vi "Remove NaN-containing Pairs.vi"(8 "Error In":errorcluster, 9 "Y Array in":dbl[](array[numeric]), 10 "Elements to remove (NaN)":dbl[](array[numeric])=[nan], 11 "X Array in":dbl[](array[numeric])) -> (0 "Error Out":errorcluster, 1 "Y Array out":dbl[](array[numeric]), 2 "# X elts deleted":i32, 3 "X Array out":dbl[](array[numeric]), 4 "Deleted Elts Indices":i32[](array[numeric]))   [LabVIEW 2021, in "Arrays.lvlib"]
uses:
  Arrays.lvlib
  <userlib>/_OpenG.lib/array/array.llb/Search 1D Array (DBL)__ogtk.vi
  <userlib>/_OpenG.lib/array/array.llb/Sort 1D Array (I32)__ogtk.vi
  <userlib>/_OpenG.lib/array/array.llb/Remove Duplicates from 1D Array (I32)__ogtk.vi
  <userlib>/_OpenG.lib/array/array.llb/Delete Elements from 1D Array (DBL)__ogtk.vi
  <userlib>/_OpenG.lib/array/array.llb/openg_array.lvlib
panel:
  out "# Y elts deleted":i32
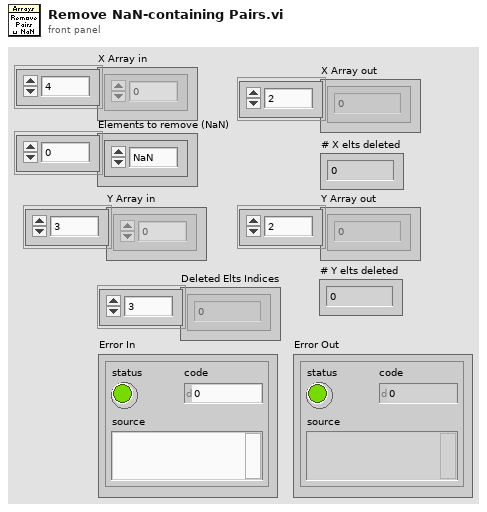
[diagram p1: front panel]
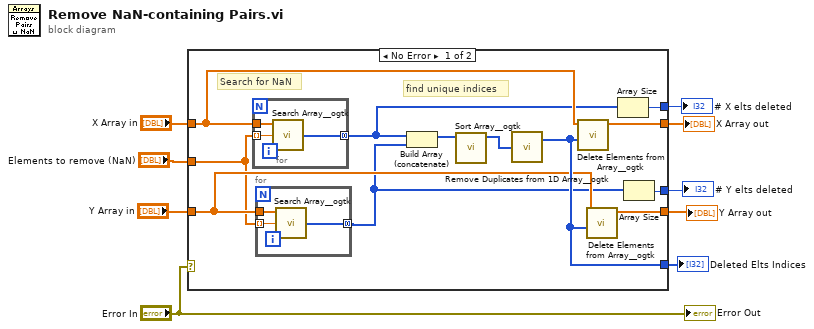
[diagram p0: block diagram]
diagram:
  n1 = case shown="No Error" "Error In" {
    tunnel: "X Array in" -> [w15 w29]
    tunnel: [w20 w29] -> w8
    tunnel: "Y Array in" -> [w13 w28]
    tunnel: [w19 w28] -> w6
    tunnel: [w18 _] -> w5
    tunnel: [w17 _] -> w4
    tunnel: [w16 _] -> w2
    tunnel: "Elements to remove (NaN)" -> [w12 _]
    frame No Error {
      # "find unique indices"
      # "Search for NaN"
      n2 = for {
        tunnel: w15 -> [w27]
        tunnel: [w25] -> w11 mode=concatenating
        tunnel: w12 -> [w26] mode=indexing
        n3 = call-poly <userlib>:"Search Array__ogtk.vi"("Array"=w27, "Element Data"=w26) -> ("Indices of Elements"=w25:i32[])  [unwired: 7 in]
      }
      n4 = for {
        tunnel: w13 -> [w24]
        tunnel: [w22] -> w10 mode=concatenating
        tunnel: w12 -> [w23] mode=indexing
        n5 = call-poly <userlib>:"Search Array__ogtk.vi"("Array"=w24, "Element Data"=w23) -> ("Indices of Elements"=w22:i32[])  [unwired: 7 in]
      }
      n6 = Build Array (concatenate)(w11, w10) -> (w14:i32[])
      n7 = call-poly <userlib>:"Sort Array__ogtk.vi"("Array in"=w14) -> ("Sorted Array out"=w21:i32[])  [unwired: 9 in, 1 out]
      n8 = call-poly <userlib>:"Remove Duplicates from 1D Array__ogtk.vi"("Input Array"=w21) -> ("Output Array"=w16:i32[])  [unwired: 1 out]
      n9 = call-poly <userlib>:"Delete Elements from Array__ogtk.vi"("indices"=w16, "array"=w15) -> ("array w/ subset deleted"=w20:dbl[])  [unwired: 8 in, 1 out]
      n10 = call-poly <userlib>:"Delete Elements from Array__ogtk.vi"("indices"=w16, "array"=w13) -> ("array w/ subset deleted"=w19:dbl[])  [unwired: 8 in, 1 out]
      n11 = Array Size(array=w11) -> (size(s)=w18:i32)
      n12 = Array Size(array=w10) -> (size(s)=w17:i32)
    }
    frame Error {
    }
  }
  "Y Array out" <- w6
  "X Array out" <- w8
  "# X elts deleted" <- w5
  "# Y elts deleted" <- w4
  "Deleted Elts Indices" <- w2
  "Error Out" <- "Error In"
